vi "test3.vi"   [LabVIEW 2012]
uses:
  <vilib>/NXT/Block Support/NXT_InputPort.ctl
  <vilib>/NXT/Dual Mode Library/Display/drawText.vi
  <vilib>/NXT/Dual Mode Library/Waits/Wait_Num(msec).vi
types:
  T1 = typedef "LVHSConnector.ctl" = cluster{"Hardware":string, "Flattened String":string}
  T2 = typedef "NXT_InputPort.ctl" = u8
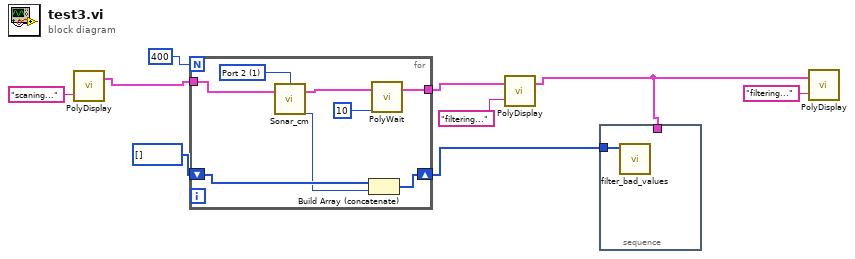
[diagram p0: block diagram]
diagram:
  n1 = call-poly <vilib>:"PolyDisplay.vi"("Text"="scaning...") -> ("NXT"=w1:T1)  [unwired: 3 in]
  n2 = for {
    N: 400 -> [_]
    shift-right: [w17] -> w7
    shift-left: i16[] [] -> [w16]
    tunnel: [w12] -> w6
    tunnel: w1 -> [w10]
    w15 = T2 1 items=["Port 1", "Port 2", "Port 3", "Port 4"] ("Port (Port 4)")
    n3 = call <vilib>:"Sonar_cm.vi"("NXT"=w10, "Port (Port 4)"=w15) -> ("Distance (cm)"=w13:i16, "NXT"=w14:T1)  [unwired: 1 in]
    n4 = Build Array (concatenate)(w16, w13) -> (w17:i16[])
    n5 = call-poly <vilib>:"PolyWait.vi"("Time (100 msec)"=10, "NXT"=w14) -> ("NXT"=w12:T1)  [unwired: 2 in]
  }
  n6 = call-poly <vilib>:"PolyDisplay.vi"("Text"="filtering...", "NXT"=w6) -> ("NXT"=w3:T1)  [unwired: 2 in]
  n7 = stacked-sequence {
    tunnel: w7 -> [w18]
    tunnel: w3 -> [_]
    frame #0 {
      n8 = call "filter_bad_values.vi"("Array 3"=w18) -> ()  [unwired: 10 in, 1 out]
    }
  }
  n9 = call-poly <vilib>:"PolyDisplay.vi"("Text"="filtering...", "NXT"=w3) -> ()  [unwired: 2 in, 1 out]
